vi "Open Connection.vi"(11 "Setup Parameters":T2) -> (0 "error out":errorcluster, 3 "AR Drone Resource":T1)   [LabVIEW 2014]
uses:
  <vilib>/LVH/AR Drone Toolkit/Type Defs/AR Drone Resource.ctl
  <vilib>/LVH/AR Drone Toolkit/AR Drone.lvlib
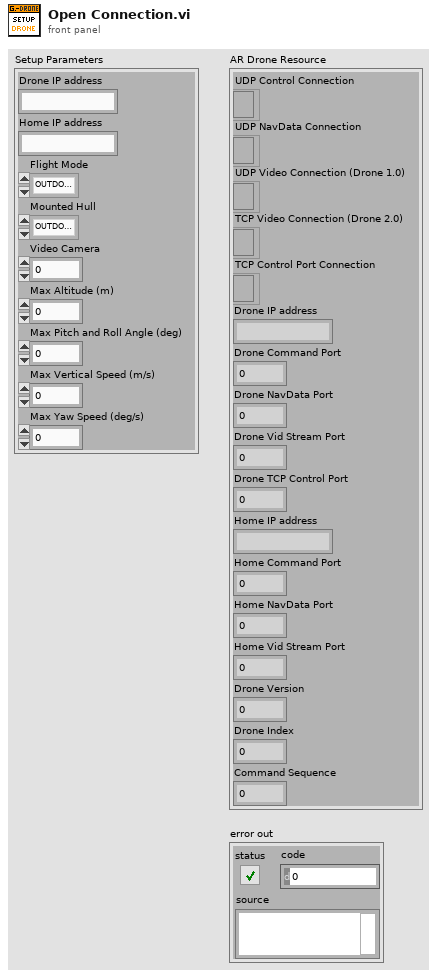
[diagram p1: front panel]
types:
  T1 = typedef "AR Drone.lvlib/AR Drone Resource.ctl" = cluster{"UDP Control Connection":refnum<k16>, "UDP NavData Connection":refnum<k16>, "UDP Video Connection (Drone 1.0)":refnum<k16>, "TCP Video Connection (Drone 2.0)":refnum<k5>, "TCP Control Port Connection":refnum<k5>, "Drone IP address":string, "Drone Command Port":u16, "Drone NavData Port":u16, "Drone Vid Stream Port":u16, "Drone TCP Control Port":u16, "Home IP address":string, "Home Command Port":u16, "Home NavData Port":u16, "Home Vid Stream Port":u16, "Drone Version":i32, "Drone Index":i32, "Command Sequence":i32}
  T2 = cluster{"Drone IP address":string, "Home IP address":string, "Flight Mode":enum8{"OUTDOOR MODE", "INDOOR MODE"}, "Mounted Hull":enum8{"OUTDOOR HULL", "INDOOR HULL"}, "Video Camera":u8, "Max Altitude (m)":sgl, "Max Pitch and Roll Angle (deg)":sgl, "Max Vertical Speed (m/s)":sgl, "Max Yaw Speed (deg/s)":sgl}
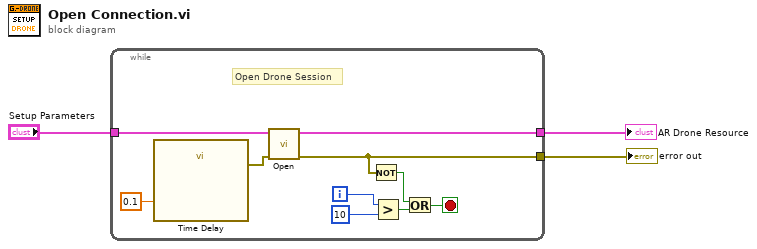
[diagram p0: block diagram]
diagram:
  n1 = while {
    tunnel: "Setup Parameters" -> [w13]
    tunnel: [w6] -> w2
    tunnel: [w5] -> w1
    i -> [w9]
    stop <- w11 stop-if-true
    # "Open Drone Session"
    n2 = call "Time Delay"("Delay Time (s)"=0.1) -> ("error out"=w7:errorcluster)  [unwired: 10 in]
    n3 = call <vilib>:"Open.vi"("error in (no error)"=w7, "Setup Parameters"=w13) -> ("error out"=w5:errorcluster, "AR Drone Resource"=w6:T1)  [unwired: 8 in]
    n4 = Not(x=w5) -> (.not. x?=w4:bool)
    n5 = Greater?(x=w9, y=10) -> (0:w10:bool)
    n6 = Or(x=w4, y=w10) -> (x .or. y?=w11:bool)
  }
  "error out" <- w1
  "AR Drone Resource" <- w2
